vi "GLdrv_MEAS_OUTP_CLR.vi"(0 "Connection ID":T1, 11 "error in (no error)":errorcluster) -> (4 "Connection ID Out":T1, 6 "Status out":string, 15 "error out":errorcluster)   [LabVIEW 2017, in "GL860_Driver.lvlib"]
doc: "リアルタイムデータ転送バッファのクリアを実行します。\n初回のACK?でデータ受け取り前にバッファをクリアしてください\n必ず“#6000000”がレスポンスされます。\n例） :MEAS:CLR? → #6000000\n※#6000000の後ろには改行コードは送信されません。\n8バイトのバイナリー受信を行ってください。"
uses:
  GL860_Driver.lvlib
  ConnectionID.ctl
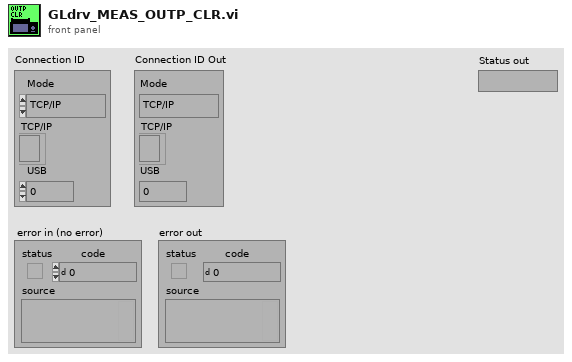
[diagram p1: front panel]
types:
  T1 = typedef "ConnectionID.ctl" = cluster{"Mode":enum16{"TCP/IP", "USB"}, "TCP/IP":refnum<k5>, "USB":i32}
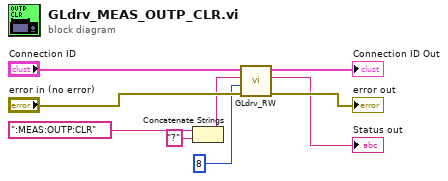
[diagram p0: block diagram]
diagram:
  n1 = Concatenate Strings(":MEAS:OUTP:CLR" ("Command"), "?" ("string")) -> (w3:string)
  n2 = call "GLdrv_RW.vi"("error in (no error)"="error in (no error)", "Count(0:[CR+LF])"=u32 8, "data in"=w3, "Connection ID"="Connection ID") -> ("error out"=→"error out":errorcluster, "data out"=→"Status out":string, "Connection ID Out"=→"Connection ID Out":T1)  [unwired: 3 in, 2 out]
